vi "Insight_Measure_Spatial_Step.vi"(8 "error in (no error)":errorcluster, 11 "telnet connection":T1) -> (0 "error out":errorcluster, 1 "response data":string, 2 "Spatial Step (mm)":dbl, 3 "telnet  connection out":T1)   [LabVIEW 2011]
doc: "Insight Photonic Solutions\n\nThis VI reads the spatial step size, in millimeters, between points in the PSF calculated by the laser in Data Streaming mode of the Measurement of User data.\n\nver 1.0 - original release"
uses:
  Telnet Session.ctl
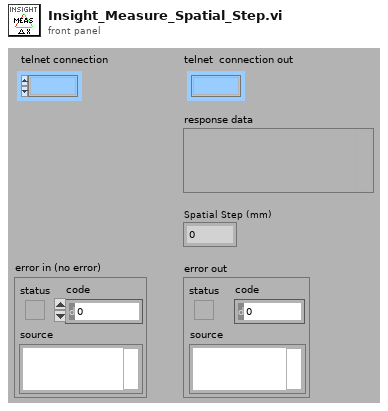
[diagram p1: front panel]
types:
  T1 = typedef "Telnet Session.ctl" = refnum<k1>
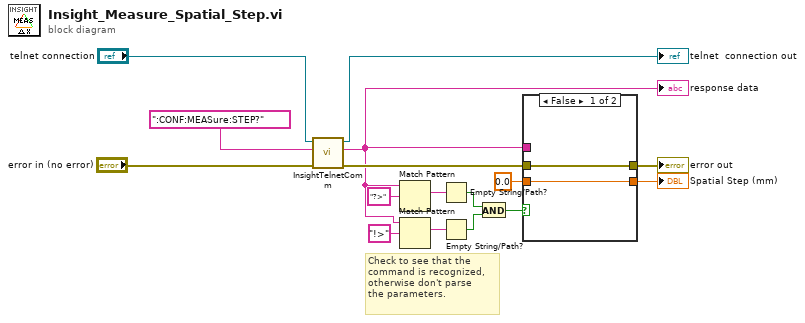
[diagram p0: block diagram]
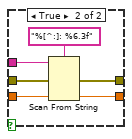
[diagram p2: hidden frame]
diagram:
  # "Check to see that the \ncommand is recognized,\notherwise don't parse \nthe parameters."
  n1 = call "InsightTelnetComm.vi"("error in"="error in (no error)", "write buffer (\"\")"=":CONF:MEASure:STEP?" ("String"), "telnet connection"="telnet connection") -> ("error out"=w15:errorcluster, "response data"=w3:string, "telnet  connection out"=→"telnet  connection out":T1)  [unwired: 4 in]
  "response data" <- w3
  n2 = Match Pattern(string=w3, regular expression="?>") -> (match substring=w8:string)  [unwired: 1 in, 3 out]
  n3 = Match Pattern(string=w3, regular expression="!>") -> (match substring=w7:string)  [unwired: 1 in, 3 out]
  n4 = Empty String/Path?(string/path=w8) -> (empty?=w5:bool)
  n5 = Empty String/Path?(string/path=w7) -> (empty?=w4:bool)
  n6 = And(x=w5, y=w4) -> (x .and. y?=w2:bool)
  n7 = case shown="False" w2 {
    tunnel: [w18 w23] -> w16
    tunnel: w15 -> [w18 w22]
    tunnel: [w17 w21] -> w10
    tunnel: w3 -> [_ w20]
    tunnel: 0.0 ("default value 1") -> [w17 w19]
    frame False {
    }
    frame True {
      n8 = Scan From String(format string="%[^:]: %6.3f", input string=w20, error in=w22, default 2=w19) -> (error out=w23:errorcluster, output 2=w21:dbl)  [unwired: 3 in, 2 out]
    }
  }
  "error out" <- w16
  "Spatial Step (mm)" <- w10
